vi "Write Session Reservation.vi"(8 "error in (no error)":errorcluster, 10 "Session Reservation":refnum<class "Session Reservation.lvclass">, 11 "DMM_Base in":refnum<class "DMM_Base.lvclass">) -> (0 "error out":errorcluster, 3 "DMM_Base out":refnum<class "DMM_Base.lvclass">)   [LabVIEW 2021, in "DMM_Base.lvclass"]
uses:
  DMM_Base.lvclass
  <vilib>/Plug-In SDKs/Clients/Session Management V1/Session Reservation/Session Reservation.lvclass
  DMM_Base.lvclass/DMM_Base.ctl
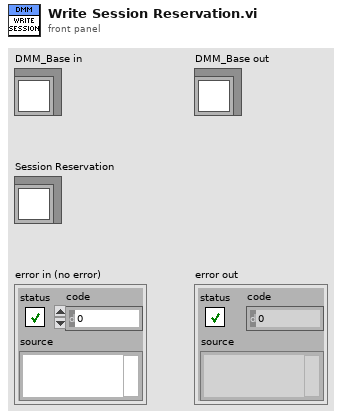
[diagram p1: front panel]
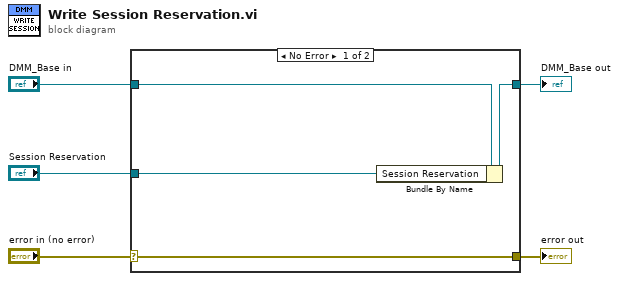
[diagram p0: block diagram]
diagram:
  n1 = case shown="No Error" "error in (no error)" {
    selector: "error in (no error)" -> [w9 w10]
    tunnel: [w9 w10] -> w4
    tunnel: [w7 w11] -> w2
    tunnel: "DMM_Base in" -> [w8 w11]
    tunnel: "Session Reservation" -> [w6 _]
    frame No Error {
      n2 = Bundle By Name(cluster=w8, "Session Reservation"=w6) -> (w7:refnum<class "DMM_Base.lvclass">)
    }
    frame Error {
    }
  }
  "error out" <- w4
  "DMM_Base out" <- w2
